vi "deleteTuplaEnDBReceta.vi"(8 "error in":errorcluster, 11 "claseReceta in":refnum<class "claseReceta.lvclass">) -> (0 "error out":errorcluster, 3 "claseReceta out":refnum<class "claseReceta.lvclass">)   [LabVIEW 2014, in "claseReceta.lvclass"]
uses:
  claseReceta.lvclass
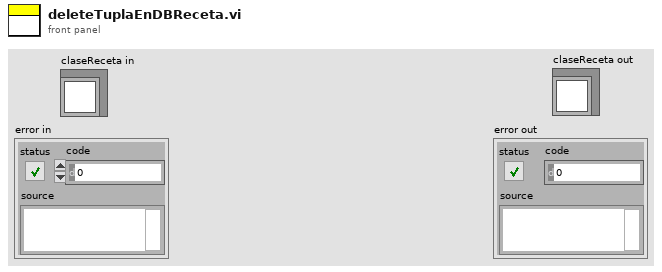
[diagram p1: front panel]
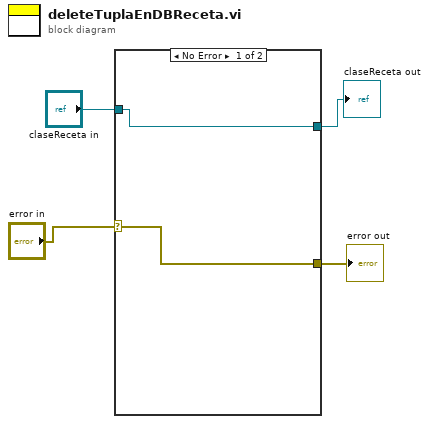
[diagram p0: block diagram]
diagram:
  n1 = case shown="No Error" "error in" {
    selector: "error in" -> [w6 w8]
    tunnel: [w6 w8] -> w3
    tunnel: [w5 w7] -> w2
    tunnel: "claseReceta in" -> [w5 w7]
    frame No Error {
    }
    frame Error {
    }
  }
  "claseReceta out" <- w2
  "error out" <- w3
